vi "Is Metronome.vi"(11 "Actor Name":string) -> (3 "Is Metronome":bool)   [LabVIEW 2015, in "Actor.lvclass"]
uses:
  Actor.lvclass
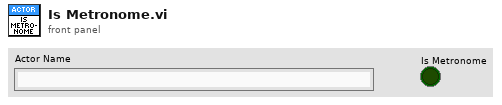
[diagram p1: front panel]
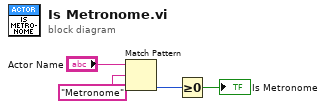
[diagram p0: block diagram]
diagram:
  n1 = Match Pattern(string="Actor Name", regular expression="Metronome") -> (offset past match=w2:i32)  [unwired: 1 in, 3 out]
  n2 = Greater Or Equal To 0?(x=w2) -> (x >= 0?=→"Is Metronome":bool)
